vi "Pack Step Value.vi"(8 "error in":errorcluster, 10 "Value":string, 11 "Message Step in":refnum<class "Message Step.lvclass">) -> (0 "error out":errorcluster, 3 "Message Step out":refnum<class "Message Step.lvclass">)   [LabVIEW 2017, in "Controller.lvlib" / "Message Step.lvclass"]
uses:
  Message Step.lvclass
  Message Step.lvclass/Message Step.ctl
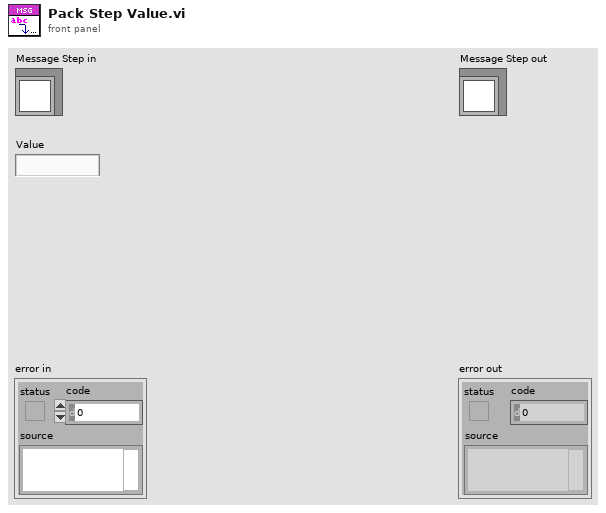
[diagram p1: front panel]
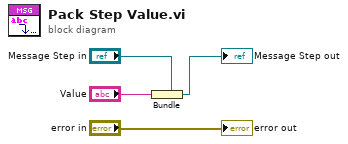
[diagram p0: block diagram]
diagram:
  n1 = Bundle(cluster="Message Step in", "Value") -> (→"Message Step out":refnum<class "Message Step.lvclass">)
  "error out" <- "error in"
